vi "change alarm comparison operation.vi"(5 "Limit":dbl, 7 "comparison":T1, 8 "error in":errorcluster, 9 "compare index":i32, 10 "alarm name":string, 11 "alarms module configuration in":refnum<class "alarms module configuration.lvclass">) -> (0 "error out":errorcluster, 3 "alarms module configuration out":refnum<class "alarms module configuration.lvclass">)   [LabVIEW 2013, in "alarms module configuration.lvclass"]
uses:
  alarms module configuration.lvclass
  compare type.ctl
  alarms module configuration.lvclass/alarms module configuration.ctl
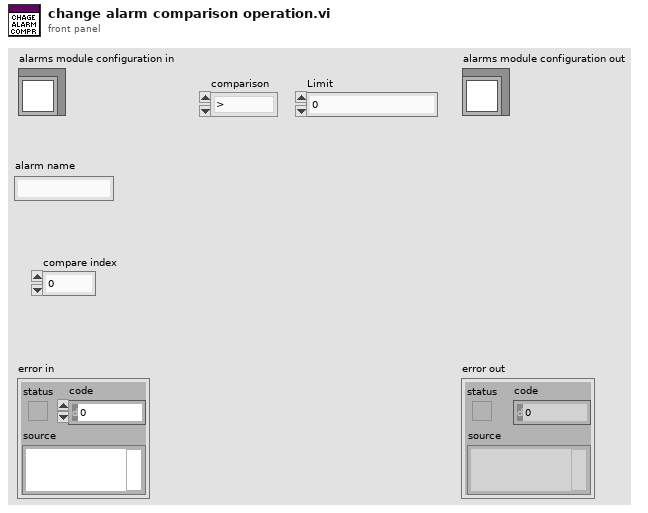
[diagram p1: front panel]
types:
  T1 = typedef "alarms module configuration.lvclass/compare type.ctl" = enum16{">", "<", ">=", "<=", "="}
  T2 = typedef "alarms module configuration.lvclass/alarm configuration.ctl" = cluster{"alarm name":string, "comparisons":T3[], "unlatch":refnum<class "TBM channel.lvclass">, "output":refnum<class "TBM channel.lvclass">, "boolean op":T4}
  T3 = typedef "alarms module configuration.lvclass/alarm comparison.ctl" = cluster{"input channel":refnum<class "TBM channel.lvclass">, "limit":dbl, "comparison":T1}
  T4 = typedef "alarms module configuration.lvclass/boolean operation.ctl" = enum16{"AND", "OR"}
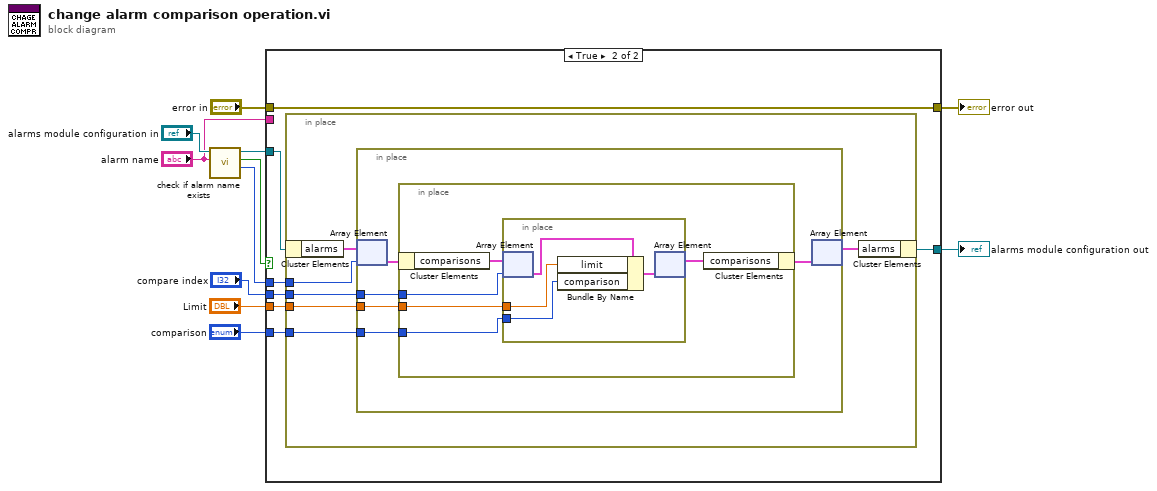
[diagram p0: block diagram]
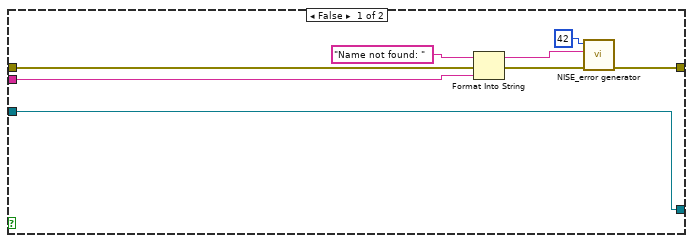
[diagram p2: hidden frame]
diagram:
  n1 = call "check if alarm name exists.vi"("name to locate"="alarm name", "alarms module configuration in"="alarms module configuration in") -> ("index"=w5:i32, "found?"=w8:bool, "alarms module configuration out"=w6:refnum<class "alarms module configuration.lvclass">)  [unwired: 6 in, 1 out]
  n2 = case shown="True" w8 {
    tunnel: [w18 w24] -> w10
    tunnel: "error in" -> [w19 w24]
    tunnel: [w13 w25] -> w7
    tunnel: w6 -> [w13 w26]
    tunnel: w5 -> [_ w23]
    tunnel: "alarm name" -> [w12 _]
    tunnel: "compare index" -> [_ w22]
    tunnel: "Limit" -> [_ w21]
    tunnel: "comparison" -> [_ w20]
    frame False {
      n3 = Format Into String(initial string="Name not found: " ("append error message"), error in=w19, w12) -> (resulting string=w14:string, error out=w16:errorcluster)  [unwired: 1 in]
      n4 = call <vilib>:"NISE_error generator.vi"("error in"=w16, "append error message"=w14, "error code (0)"=42) -> ("error out"=w18:errorcluster)  [unwired: 6 in]
    }
    frame True {
      n5 = in-place {
        in-place-border: w23 -> [w30]
        in-place-border: w22 -> [w29]
        in-place-border: w21 -> [w28]
        in-place-border: w20 -> [w27]
        n6 = in-place-cluster #1(w26) -> ("alarms"=w32:T2[])
        n7 = in-place {
          in-place-border: w29 -> [w36]
          in-place-border: w28 -> [w35]
          in-place-border: w27 -> [w34]
          n8 = in-place-array #2(w32, w30) -> (w37:T2)
          n9 = in-place {
            in-place-border: w36 -> [w40]
            in-place-border: w35 -> [w39]
            in-place-border: w34 -> [w38]
            n10 = in-place-cluster #3(w37) -> ("comparisons"=w42:T3[])
            n11 = in-place {
              in-place-border: w39 -> [w44]
              in-place-border: w38 -> [w43]
              n12 = in-place-array #4(w42, w40) -> (w46:T3)
              n13 = Bundle By Name(cluster=w46, "limit"=w44, "comparison"=w43) -> (w45:T3)
              n14 = in-place-array #4(w45) -> (w41:T3[])  [unwired: 1 out]
            }
            n15 = in-place-cluster #3("comparisons"=w41) -> (w33:T2)
          }
          n16 = in-place-array #2(w33) -> (w31:T2[])  [unwired: 1 out]
        }
        n17 = in-place-cluster #1("alarms"=w31) -> (w25:refnum<class "alarms module configuration.lvclass">)
      }
    }
  }
  "error out" <- w10
  "alarms module configuration out" <- w7
